vi "Set Voltage SP.vi"(8 "error in (no error)":errorcluster, 10 "Voltage SP":dbl format="%.2f", 11 "VISA session":refnum<visa-resource-name>) -> (0 "error out":errorcluster, 3 "dup VISA session":refnum<visa-resource-name>)   [LabVIEW 2011, in "Magna PSU.lvlib"]
uses:
  Magna PSU.lvlib
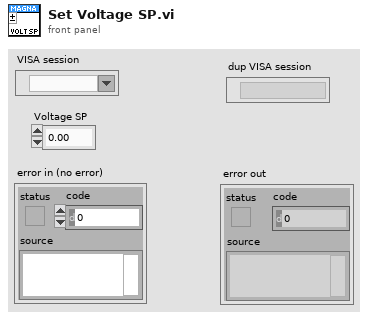
[diagram p1: front panel]
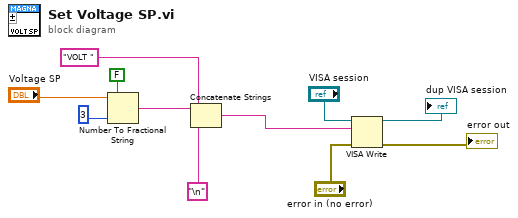
[diagram p0: block diagram]
diagram:
  n1 = Number To Fractional String(use system decimal point (T)=FALSE, number="Voltage SP", precision (6)=3) -> (F-format string=w6:string)  [unwired: 1 in]
  n2 = Concatenate Strings("VOLT ", w6, "\n") -> (w1:string)
  n3 = VISA Write(VISA resource name="VISA session", write buffer=w1, error in (no error)="error in (no error)") -> (VISA resource name out=→"dup VISA session":refnum<visa-resource-name>, error out=→"error out":errorcluster)  [unwired: 1 out]
